vi "Update-control-references.vi"(8 "error in (no error)":errorcluster, 11 "VI Reference":refnum<vi>) -> (0 "error out":errorcluster, 2 "Control refs":refnum<vi>[](array[refnum]), 3 "VI Reference":refnum<vi>)   [LabVIEW 2013, in "HardwareCharacterization.lvlib" / "HC-UI.lvclass"]
uses:
  HC-UI.lvclass
  Control-names.ctl
panel:
  in  "Control names":T1
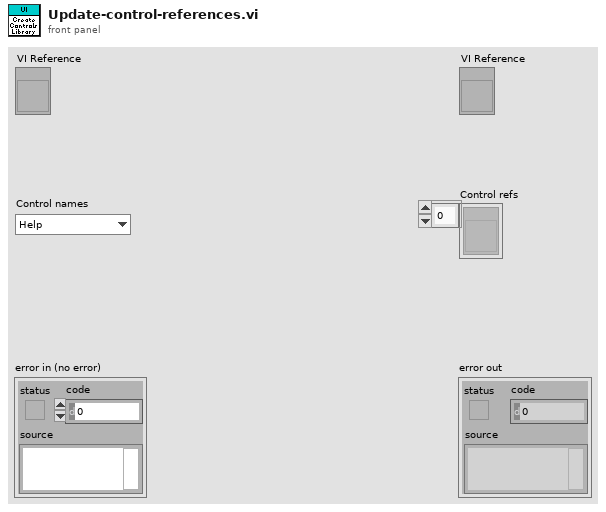
[diagram p1: front panel]
types:
  T1 = typedef "HardwareCharacterization.lvlib/HC-UI.lvclass/Control-names.ctl" = enum16{"Help", "Status", "Load configuration", "Save configuration", "Activate", "Start", "Stop", "Options"}
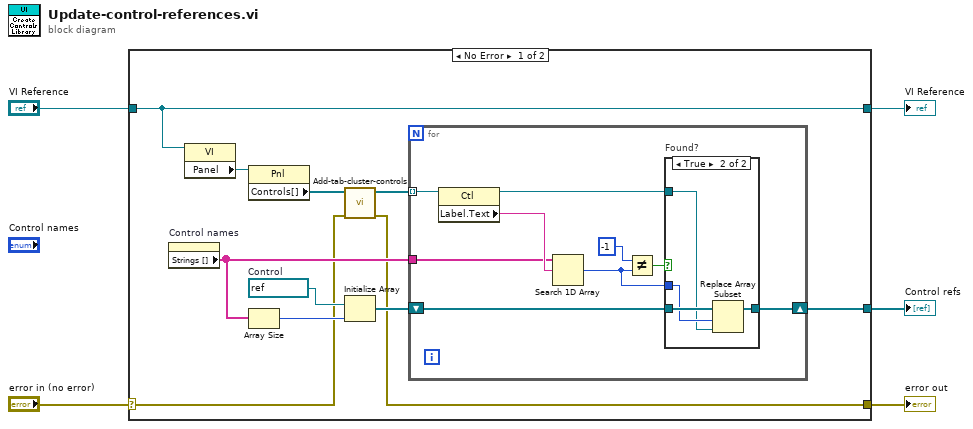
[diagram p0: block diagram]
diagram:
  n1 = case shown="No Error" "error in (no error)" {
    selector: "error in (no error)" -> [w7 w32]
    tunnel: [w6 w32] -> w4
    tunnel: [w10 w31] -> w2
    tunnel: "VI Reference" -> [w10 w31]
    tunnel: [w11 _] -> w1
    frame No Error {
      w14 = refnum<vi> refnum  # Control
      n2 = property on="Control names" class="Enum (strict)"() -> ("Strings []"=w12:string[])  [unwired: 2 in, 2 out]
      n3 = property class="VI"(reference=w10) -> ("Panel"=w16:refnum<vi>)  [unwired: 1 in, 2 out]
      n4 = property class="Pnl"(reference=w16) -> ("Controls[]"=w9:refnum<vi>[])  [unwired: 1 in, 2 out]
      n5 = Array Size(array=w12) -> (size(s)=w15:i32)
      n6 = call "Add-tab-cluster-controls.vi"("error in (no error)"=w7, "Controls in"=w9) -> ("error out"=w6:errorcluster, "Controls out"=w8:refnum<vi>[])  [unwired: 8 in]
      n7 = Initialize Array(w14, w15) -> (w13:refnum<vi>[])
      n8 = for {
        tunnel: w8 -> [w25] mode=indexing
        tunnel: w12 -> [w23]
        shift-right: [w19] -> w11
        shift-left: w13 -> [w20]
        n9 = property class="Ctl"(reference=w25) -> (reference out=w18:refnum<vi>, "Label.Text"=w24:string)  [unwired: 1 in, 1 out]
        n10 = Search 1D Array(1D array=w23, element=w24) -> (index of element=w17:i32)  [unwired: 1 in]
        n11 = Not Equal?(x=-1, y=w17) -> (x != y?=w21:bool)
        n12 = case "Found?" shown="True" w21 {
          tunnel: w20 -> [w26 w30]
          tunnel: [w26 w29] -> w19
          tunnel: w18 -> [_ w27]
          tunnel: w17 -> [_ w28]
          frame False {
          }
          frame True {
            n13 = Replace Array Subset(array=w30, new element=w27, index=w28) -> (w29:refnum<vi>[])
          }
        }
      }
    }
    frame Error {
    }
  }
  "error out" <- w4
  "VI Reference" <- w2
  "Control refs" <- w1
